vi "test Bad Regex.vi"(8 "error in":errorcluster) -> (0 "error out":errorcluster)   [LabVIEW 2020, in "ase.test.lvlib"]
uses:
  ase.test.lvlib
  ase/ase/Configuration.ctl
  ase/ase/Windows UTF8 Conversion Mode.ctl
  ase/ase/ase.lvclass/ase.ctl
  ase/ase/Trim Whitespace.vi
  ase/ase/Merge Call Library Errors.vi
  ase/ase/Check Shared Library Version.vi
  ase/ase/Start Call.vi/a70fc713-9ee9-4497-bede-7e71c94245f2.vi
  ase/ase/Error Invalid ASE Handle.vi
  ase/ase/Error Internal Library Implementation Error.vi
  <vilib>/Utility/file.llb/Application Directory.vi
  <vilib>/Utility/error.llb/Error Cluster From Error Code.vi
  ase/ase/Wait on Call.vi
  <vilib>/addons/_JKI Toolkits/Caraya/classes/Assert/Assert Equal Value and Type_Variant.vi
  ase/ase/ase.lvclass
  <vilib>/addons/_JKI Toolkits/Caraya/classes/Test/Test.lvclass
  <vilib>/addons/_JKI Toolkits/Caraya/classes/Assert/Assert.lvclass
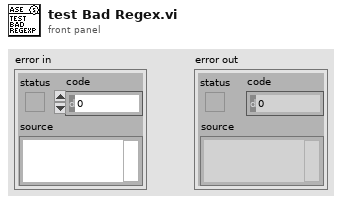
[diagram p1: front panel]
types:
  T1 = typedef "ase.lvlib/ase.lvclass/Configuration.ctl" = cluster{"Std Out Stream-Split RegExp Pattern":string, "Std Err Stream-Split RegExp Pattern":string, "ID":string, "Windows UTF8 Conversion":T2}
  T2 = typedef "ase.lvlib/ase.lvclass/Windows UTF8 Conversion Mode.ctl" = enum8{"None (Pass Through UTF8)", "To ACP Code Page", "To OEM Code Page"}
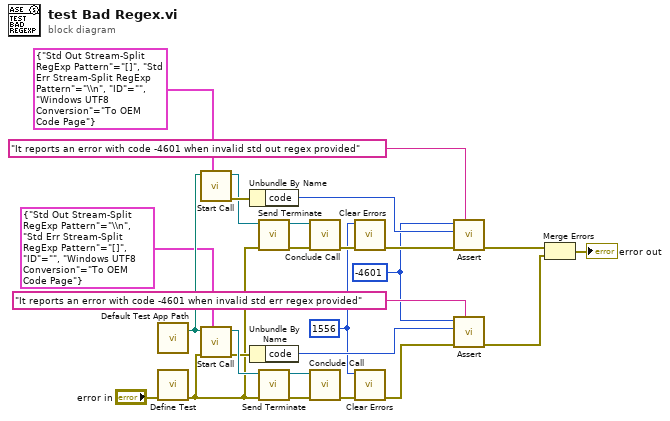
[diagram p0: block diagram]
diagram:
  w3 = 1556
  w5 = -4601 ("code")
  n1 = call "Default Test App Path.vi"() -> ("Exe Path With Extention"=w4:path)  [unwired: 2 in, 1 out]
  n2 = call <vilib>:"Define Test.vi"("error in (no error)"="error in") -> ("error out"=w6:errorcluster)  [unwired: 9 in, 1 out]
  n3 = call "Start Call.vi"("Configuration (Default)"=T1 {"Std Out Stream-Split RegExp Pattern"="[]", "Std Err Stream-Split RegExp Pattern"="\\n", "ID"="", "Windows UTF8 Conversion"=enum."To OEM Code Page"}, "Executable Path"=w4) -> ("error out"=w18:errorcluster, "New ASE Handle"=w17:refnum<class "ase.lvclass">)  [unwired: 8 in]
  n4 = call "Start Call.vi"("Configuration (Default)"=T1 {"Std Out Stream-Split RegExp Pattern"="\\n", "Std Err Stream-Split RegExp Pattern"="[]", "ID"="", "Windows UTF8 Conversion"=enum."To OEM Code Page"}, "error in"=w6, "Executable Path"=w4) -> ("error out"=w15:errorcluster, "New ASE Handle"=w16:refnum<class "ase.lvclass">)  [unwired: 7 in]
  n5 = Unbundle By Name(w18) -> ("code"=w24:i32)
  n6 = Unbundle By Name(w15) -> ("code"=w10:i32)
  n7 = call "Send Terminate.vi"("error in"=w6, "ASE Handle"=w17) -> ("error out"=w19:errorcluster, "ASE Handle Duplicate"=w20:refnum<class "ase.lvclass">)  [unwired: 7 in, 1 out]
  n8 = call "Send Terminate.vi"("error in"=w6, "ASE Handle"=w16) -> ("error out"=w14:errorcluster, "ASE Handle Duplicate"=w13:refnum<class "ase.lvclass">)  [unwired: 7 in, 1 out]
  n9 = call "Conclude Call.vi"("error in"=w19, "ASE Handle"=w20) -> ("error out"=w23:errorcluster)  [unwired: 7 in, 2 out]
  n10 = call "Conclude Call.vi"("error in"=w14, "ASE Handle"=w13) -> ("error out"=w11:errorcluster)  [unwired: 7 in, 2 out]
  n11 = call <vilib>:"Clear Errors.vi"("error in (no error)"=w23, "specific error code to clear (0: all)"=w3) -> ("error out"=w21:errorcluster)  [unwired: 4 in, 1 out]
  n12 = call <vilib>:"Clear Errors.vi"("error in (no error)"=w11, "specific error code to clear (0: all)"=w3) -> ("error out"=w12:errorcluster)  [unwired: 4 in, 1 out]
  n13 = call-poly <vilib>:"Assert.vi"("Label"="It reports an error with code -4601 when invalid std out regex provided", "error in (no error)"=w21, "Y"=w24, "X"=w5) -> ("error out"=w22:errorcluster)  [unwired: 6 in, 1 out]
  n14 = call-poly <vilib>:"Assert.vi"("Label"="It reports an error with code -4601 when invalid std err regex provided", "error in (no error)"=w12, "Y"=w10, "X"=w5) -> ("error out"=w8:errorcluster)  [unwired: 6 in, 1 out]
  n15 = Merge Errors(w22, w8) -> (→"error out":errorcluster)
